vi "Main.vi"(11 "Module Admin":refnum<class "Delacor_lib_QMH_Module Admin.lvclass">) -> ()   [LabVIEW 2022 SP3, in "Server.lvlib"]
doc: "This template is based off of the Queued Message Handler design pattern and the Queued Message Handler project template that ships with LabVIEW.\n\nThe main difference is that the queue is private to this module and communication between modules is performed via Broadcast and Request events.\n\nRequest events are wrapped in public API methods and are handled in the Event Handling Loop (EHL) of this VI. Any module can register for Broadcast events sent by this module. The EHL generates messages based on user interface actions.\n\nThe Message Handling Loop (MHL) processes messages generated by the EHL, or by other messages. The messages are string values, so new messages can be added easily to the Message Cases case structure in the MHL. Each message cluster can also provide an optional value for Message Data, which is a variant that can be converted to whatever message-specific data is required.\n_____\nBased on DQMH Project Template 6.1.0.94."
uses:
  Server.lvlib
  <vilib>/Delacor/Delacor QMH/Libraries/Module Admin_class/Delacor_lib_QMH_Module Admin.lvclass
  Module Data--cluster.ctl
  <vilib>/Delacor/Delacor QMH/Libraries/Message Queue_class/Delacor_lib_QMH_Message Queue.lvclass/Delacor_lib_QMH_Message Queue.ctl
  Stop Argument--cluster.ctl
  <vilib>/Delacor/Delacor QMH/Libraries/Module Admin_class/Delacor_lib_QMH_Module Admin.lvclass/Delacor_lib_QMH_Module Admin.ctl
  <vilib>/Utility/miscctls.llb/LVPointTypeDef.ctl
  <vilib>/Delacor/Delacor QMH/Libraries/Message Queue_class/Delacor_lib_QMH_Enqueue Message (Single).vi
  <vilib>/Delacor/Delacor QMH/Libraries/Module Admin_class/Delacor_lib_QMH_Get External Launch.vi
  <vilib>/Utility/error.llb/Error Cluster From Error Code.vi
  <vilib>/ErrorRing/Error Ring.xnode
  <vilib>/Delacor/Delacor QMH/Libraries/Message Queue_class/Delacor_lib_QMH_Message Queue.lvclass
  User 1/User 1.lvlib
  User 2/User 2.lvlib
panel:
  in  "Launch User 2":bool
  out "error out":errorcluster
  out "Status":string
  in  "Simulate MHL Error":bool
  in  "Simulate EHL Error":bool
  # "Other QMH Modules communicate with this Module via its Public API (wrappers for its Request Events).\n\nThis Module communicates with other Modules via its Broadcast Events.\nAny module that wants to get these messages, just registers for this module's Broadcast events."
  # "This template is for the Delacor Modified Queued Message Handler design pattern.\n\nSee the block diagram for more information on how to use this template."
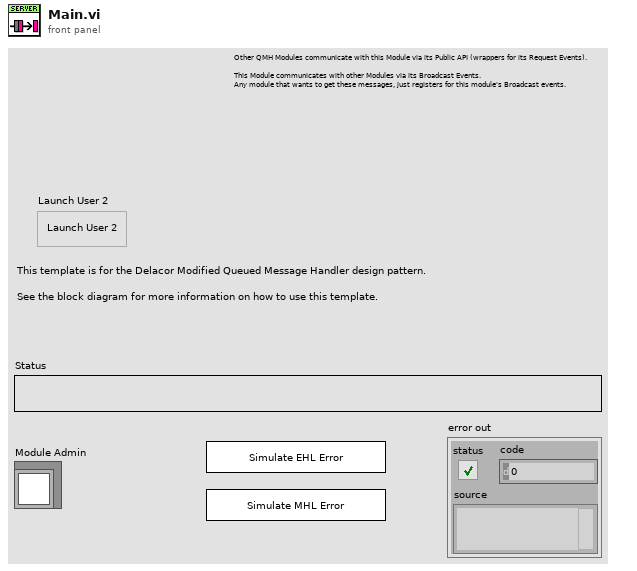
[diagram p1: front panel]
types:
  T1 = typedef "Server.lvlib/Request Events--cluster.ctl" = cluster{"Stop Module":refnum<user-event>, "Show Panel":refnum<user-event>, "Hide Panel":refnum<user-event>, "Get Module Execution Status":refnum<user-event>, "Show Diagram":refnum<user-event>}
  T2 = typedef "User 1.lvlib/Broadcast Events--cluster.ctl" = cluster{"Module Did Init":refnum<user-event>, "Status Updated":refnum<user-event>, "Error Reported":refnum<user-event>, "Module Did Stop":refnum<user-event>, "Update Module Execution Status":refnum<user-event>, "Message was sent":refnum<user-event>}
  T3 = typedef "User 2.lvlib/Broadcast Events--cluster.ctl" = cluster{"Module Did Init":refnum<user-event>, "Status Updated":refnum<user-event>, "Error Reported":refnum<user-event>, "Module Did Stop":refnum<user-event>, "Update Module Execution Status":refnum<user-event>, "Message was sent":refnum<user-event>}
  T4 = typedef "Server.lvlib/Module Data--cluster.ctl" = cluster{"Status":string}
  T5 = enum32{"invalid lock state", "Not Locked", "Locked (No Password)", "Password-protected"}
  T6 = typedef "Server.lvlib/Stop Argument--cluster.ctl" = cluster{"Origin":string, "Exit via Stop Module Req?":bool, "Wait for Module to stop?":bool}
  T7 = typedef "LVPointTypeDef.ctl" = cluster{"Horizontal":i16, "Vertical":i16}
  T8 = enum32{"Invalid", "Standard", "Closed", "Hidden", "Minimized", "Maximized"}
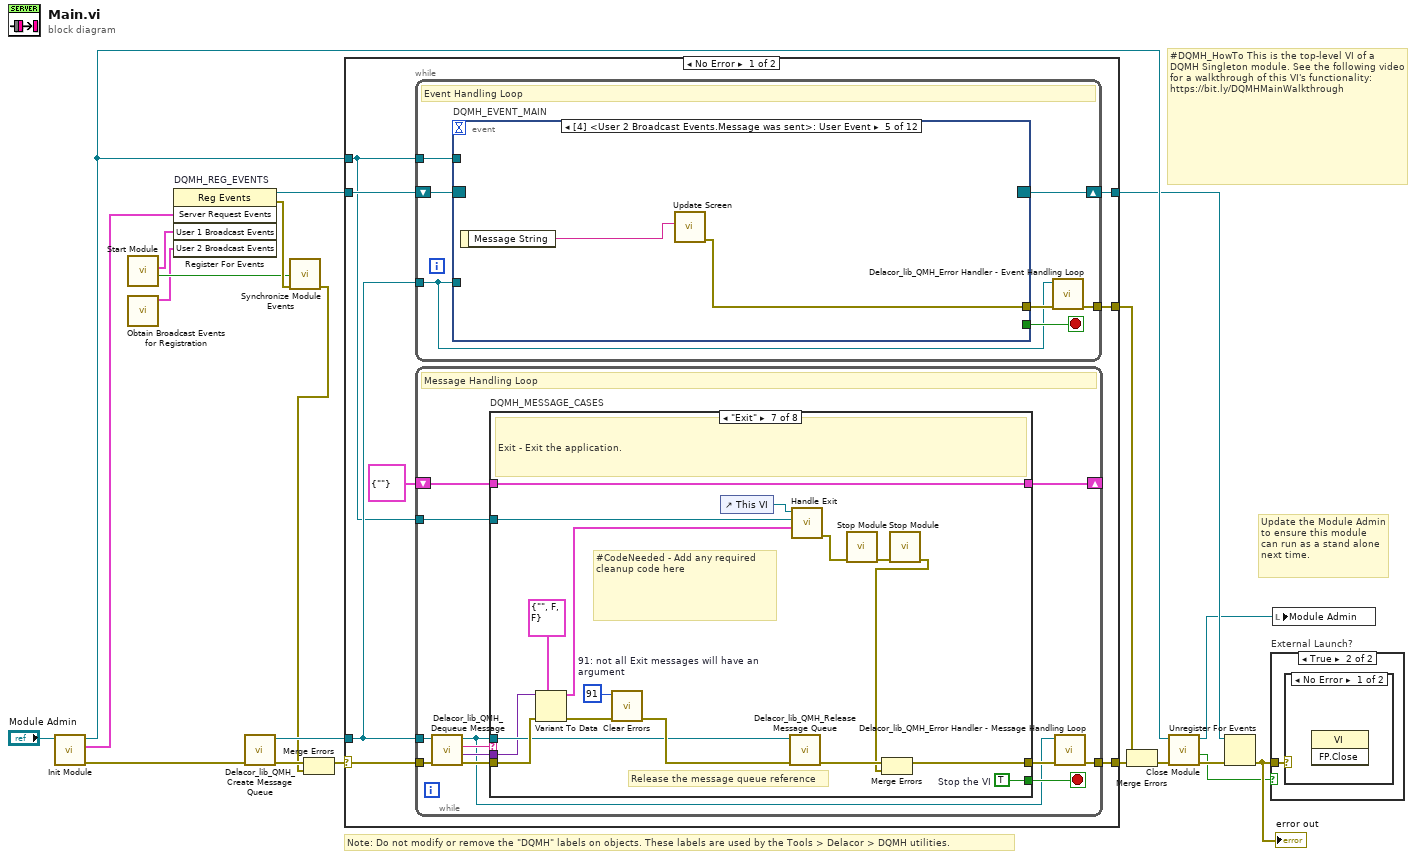
[diagram p0: block diagram]
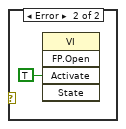
[diagram p3: hidden frame]
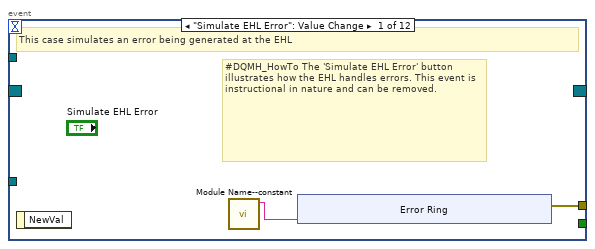
[diagram p4: hidden frame]
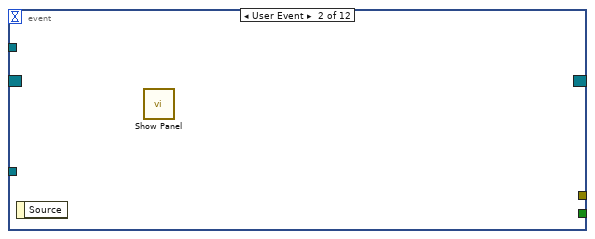
[diagram p5: hidden frame]
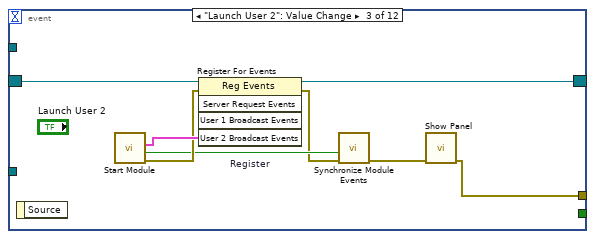
[diagram p6: hidden frame]
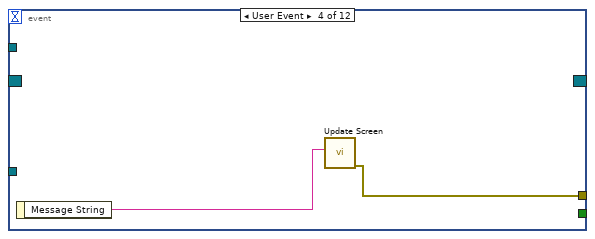
[diagram p7: hidden frame]
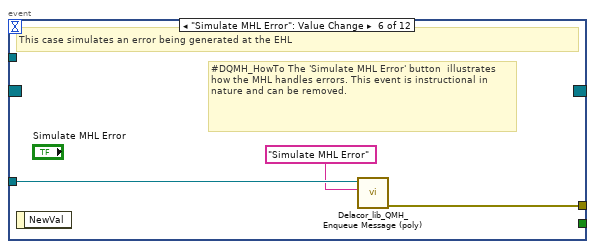
[diagram p8: hidden frame]
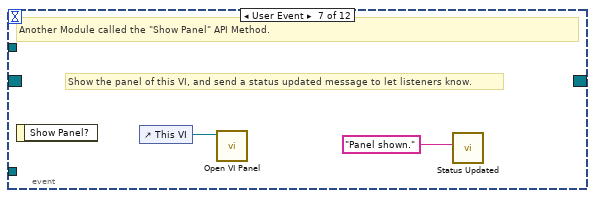
[diagram p9: hidden frame]
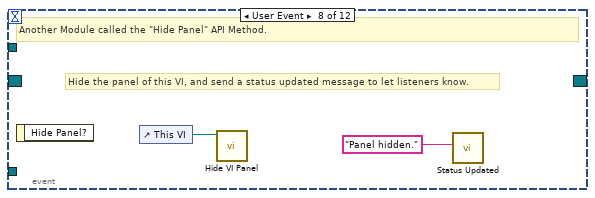
[diagram p10: hidden frame]
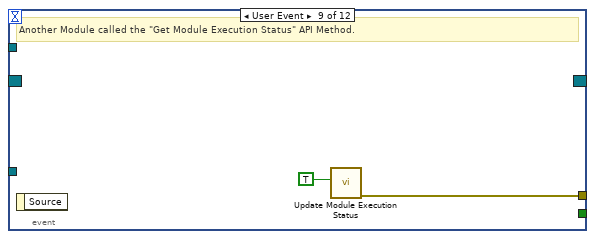
[diagram p11: hidden frame]
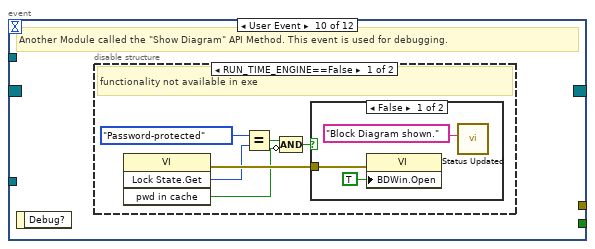
[diagram p12: hidden frame]
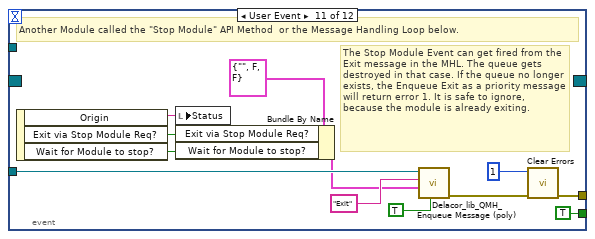
[diagram p15: hidden frame]
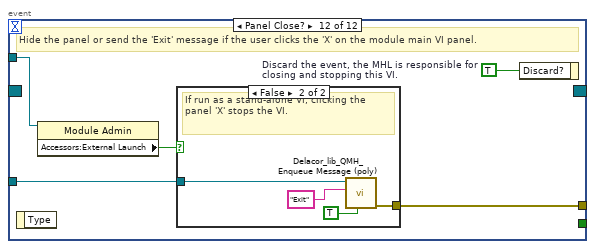
[diagram p16: hidden frame]
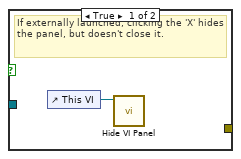
[diagram p17: hidden frame]
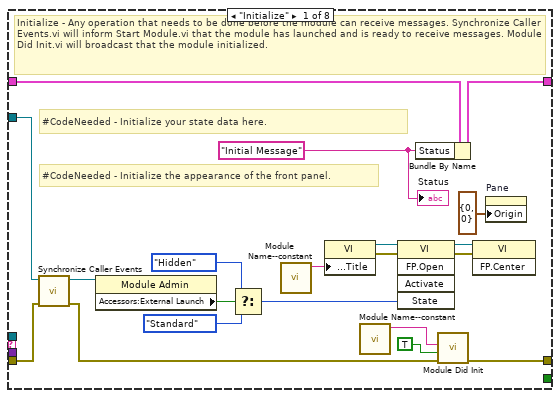
[diagram p18: hidden frame]
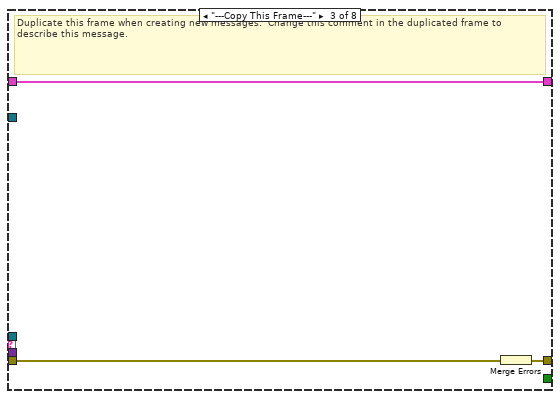
[diagram p20: hidden frame]
diagram:
  # "#DQMH_HowTo This is the top-level VI of a DQMH Singleton module. See the following video for a walkthrough of this VI's functionality: https://bit.ly/DQMHMainWalkthrough"
  # "Note: Do not modify or remove the \"DQMH\" labels on objects. These labels are used by the Tools > Delacor > DQMH utilities."
  # "Update the Module Admin to ensure this module can run as a stand alone next time."
  n1 = call "Init Module.vi"("Singleton Module Admin in"="Module Admin") -> ("error out"=w20:errorcluster, "Server Request Events"=w10:T1, "Singleton Module Admin out"=w13:refnum<class "Delacor_lib_QMH_Module Admin.lvclass">)  [unwired: 8 in]
  n2 = call "Start Module.vi"() -> ("Wait for Event Sync?"=w2:bool, "User 1 Broadcast Events"=w5:T2)  [unwired: 8 in, 2 out]
  n3 = call "Obtain Broadcast Events for Registration.vi"() -> ("User 2 Broadcast Events"=w1:T3)  [unwired: 9 in, 2 out]
  n4 = register-events "DQMH_REG_EVENTS"(w10, w5, w1) -> (reference out=w11:refnum<event-registration>, error out=w4:errorcluster)  [unwired: 2 in]
  n5 = call <vilib>:"Delacor_lib_QMH_Create Message Queue.vi"("error in"=w20) -> ("error out"=w15:errorcluster, "Message Queue"=w9:refnum<class "Delacor_lib_QMH_Message Queue.lvclass">)  [unwired: 9 in]
  n6 = call "Synchronize Module Events.vi"("error in"=w4, "Wait for Event Sync?"=w2) -> ("error out"=w3:errorcluster)  [unwired: 9 in]
  n7 = Merge Errors(w15, w3) -> (w14:errorcluster)
  n8 = case shown="No Error" w14 {
    selector: w14 -> [w27 w198]
    tunnel: [w29 w197] -> w21
    tunnel: [w26 w203] -> w12
    tunnel: w11 -> [w24 w203]
    tunnel: w9 -> [w23 w196]
    tunnel: [w28 _] -> w18
    tunnel: w13 -> [w22 w199]
    frame No Error {
      n9 = while {
        tunnel: w23 -> [w30]
        shift-right: [w33] -> w26
        shift-left: w24 -> [w34]
        tunnel: [w35] -> w28
        tunnel: w22 -> [w31]
        stop <- w32 stop-if-true
        # "Event Handling Loop"
        n10 = event "DQMH_EVENT_MAIN" shown="[4] <User 2 Broadcast Events.Message was sent>: User Event" {
          selector: w34 -> [_ _ w53 _ _ _ _ _ _ _ _ _]
          dyn-events: [_ _ w52 _ _ _ _ _ _ _ _ _] -> w33
          timeout: _ -> [_ _ _ _ _ _ _ _ _ _ _ _]
          tunnel: [_ _ _ _ _ _ _ _ _ _ TRUE ("Discard?") _] -> w32
          tunnel: w30 -> [_ _ _ _ _ w59 _ _ _ _ w83 w90]
          tunnel: [w38 _ w46 w54 w56 w60 _ _ w66 _ w86 w92] -> w36
          tunnel: w31 -> [_ _ _ _ _ _ _ _ _ _ _ w89]
          event "Simulate EHL Error": Value Change {
            # "#DQMH_HowTo The 'Simulate EHL Error' button  illustrates how the EHL handles errors. This event is instructional in nature and can be removed."
            # "This case simulates an error being generated at the EHL"
            n11 = event-data() -> ()  [unwired: 1 in, 1 out]
            n12 = call "Module Name--constant.vi"() -> ("Module Name"=w37:string)  [unwired: 11 in]
            n13 = xnode "Error Ring"("parameter 0"=w37) -> ("error out"=w38:errorcluster)
          }
          event User Event {
            n14 = event-data() -> ()  [unwired: 1 in, 1 out]
            n15 = call "Show Panel.vi"() -> ()  [unwired: 11 in, 1 out]
          }
          event "Launch User 2": Value Change {
            n16 = event-data() -> ()  [unwired: 1 in, 1 out]
            n17 = call "Start Module.vi"() -> ("error out"=w50:errorcluster, "Wait for Event Sync?"=w49:bool, "User 2 Broadcast Events"=w51:T3)  [unwired: 8 in, 1 out]
            n18 = register-events "Register"(reference=w53, error in=w50, w51) -> (reference out=w52:refnum<event-registration>, error out=w48:errorcluster)  [unwired: 2 in]
            n19 = call "Synchronize Module Events.vi"("error in"=w48, "Wait for Event Sync?"=w49) -> ("error out"=w47:errorcluster)  [unwired: 9 in]
            n20 = call "Show Panel.vi"("error in (no error)"=w47) -> ("error out"=w46:errorcluster)  [unwired: 10 in]
          }
          event User Event {
            n21 = event-data() -> ("Message String"=w55:string)  [unwired: 1 in]
            n22 = call "Update Screen.vi"("Message"=w55) -> ("error out"=w54:errorcluster)  [unwired: 10 in]
          }
          event User Event {
            n23 = event-data() -> ("Message String"=w57:string)  [unwired: 1 in]
            n24 = call "Update Screen.vi"("Message"=w57) -> ("error out"=w56:errorcluster)  [unwired: 10 in]
          }
          event "Simulate MHL Error": Value Change {
            # "#DQMH_HowTo The 'Simulate MHL Error' button  illustrates how the MHL handles errors. This event is instructional in nature and can be removed."
            # "This case simulates an error being generated at the EHL"
            n25 = event-data() -> ()  [unwired: 1 in, 1 out]
            n26 = call-poly <vilib>:"Delacor_lib_QMH_Enqueue Message (poly).vi"("Message"="Simulate MHL Error", "Message Queue in"=w59) -> ("error out"=w60:errorcluster)  [unwired: 8 in, 1 out]
          }
          event User Event {
            # "Show the panel of this VI, and send a status updated message to let listeners know."
            # "Another Module called the \"Show Panel\" API Method."
            n27 = event-data() -> ()  [unwired: 1 in, 1 out]
            n28 = control-ref of="This VI"() -> (w62:refnum<vi>)
            n29 = call "Open VI Panel.vi"("VI"=w62) -> ()  [unwired: 10 in, 1 out]
            n30 = call "Status Updated.vi"("Status"="Panel shown." ("format string")) -> ()  [unwired: 10 in, 1 out]
          }
          event User Event {
            # "Hide the panel of this VI, and send a status updated message to let listeners know."
            # "Another Module called the \"Hide Panel\" API Method."
            n31 = event-data() -> ()  [unwired: 1 in, 1 out]
            n32 = control-ref of="This VI"() -> (w64:refnum<vi>)
            n33 = call "Hide VI Panel.vi"("VI"=w64) -> ()  [unwired: 10 in, 1 out]
            n34 = call "Status Updated.vi"("Status"="Panel hidden." ("format string")) -> ()  [unwired: 10 in, 1 out]
          }
          event User Event {
            # "Another Module called the \"Get Module Execution Status\" API Method."
            n35 = event-data() -> ()  [unwired: 1 in, 1 out]
            n36 = call "Update Module Execution Status.vi"("Running?"=TRUE) -> ("error out"=w66:errorcluster)  [unwired: 10 in]
          }
          event User Event {
            # "Another Module called the \"Show Diagram\" API Method. This event is used for debugging."
            n37 = event-data() -> ()  [unwired: 1 in, 1 out]
            n38 = disable-structure shown="RUN_TIME_ENGINE==False" {
              frame condition #0 (active) {
                # "functionality not available in exe"
                n39 = invoke class="VI" method="Lock State.Get"() -> (error out=w72:errorcluster, "Get Lock State"=w71:T5, "pwd in cache"=w68:bool)  [unwired: 4 in, 1 out]
                n40 = Equal?(x=T5."Password-protected", y=w71) -> (x = y?=w69:bool)
                n41 = Compound Arithmetic op=AND(w69, invert w68) -> (w67:bool)
                n42 = case shown="False" w67 {
                  tunnel: w72 -> [w75 _]
                  frame False {
                    n43 = property class="VI"(error in=w75, "BDWin.Open"=TRUE ("Block Diagram Window:Open")) -> ()  [unwired: 1 in, 2 out]
                    n44 = call "Status Updated.vi"("Status"="Block Diagram shown." ("format string")) -> ()  [unwired: 10 in, 1 out]
                  }
                  frame True {
                    # "Password-protected VI, and the password is not in the cache. Do not show the diagram."
                  }
                }
              }
              frame condition #1 {
              }
            }
          }
          event User Event {
            # "The Stop Module Event can get fired from the Exit message in the MHL. The queue gets destroyed in that case. If the queue no longer exists, the Enqueue Exit as a priority message will return error 1. It is safe to ignore, because the module is already exiting."
            # "Another Module called the \"Stop Module\" API Method  or the Message Handling Loop below."
            n45 = event-data() -> ("Origin"=w82:string, "Exit via Stop Module Req?"=w78:bool, "Wait for Module to stop?"=w77:bool)  [unwired: 1 in]
            n46 = local write "Status"(w82) -> ()
            n47 = Bundle By Name(cluster=T6 {"Origin"="", "Exit via Stop Module Req?"=FALSE, "Wait for Module to stop?"=FALSE} ("Stop Argument"), "Exit via Stop Module Req?"=w78, "Wait for Module to stop?"=w77) -> (w76:T6)
            n48 = call-poly <vilib>:"Delacor_lib_QMH_Enqueue Message (poly).vi"("Priority Message? (F)"=TRUE, "Message Data"=w76, "Message"="Exit", "Message Queue in"=w83) -> ("error out"=w87:errorcluster)  [unwired: 6 in, 1 out]
            n49 = call <vilib>:"Clear Errors.vi"("error in (no error)"=w87, "specific error code to clear (0: all)"=1) -> ("error out"=w86:errorcluster)  [unwired: 4 in, 1 out]
          }
          event Panel Close? {
            w91 = TRUE  # Discard the event, the MHL is responsible for closing and stopping this VI.
            # "Hide the panel or send the 'Exit' message if the user clicks the 'X' on the module main VI panel."
            n50 = event-data() -> ()  [unwired: 1 in, 1 out]
            n51 = property class="Module Admin"(reference=w89) -> ("Accessors:External Launch"=w88:bool)  [unwired: 1 in, 2 out]
            n52 = case shown="False" w88 {
              tunnel: w90 -> [_ w96]
              tunnel: [_ w97] -> w92
              frame True {
                # "If externally launched, clicking the 'X' hides the panel, but doesn't close it."
                n53 = control-ref of="This VI"() -> (w93:refnum<vi>)
                n54 = call "Hide VI Panel.vi"("VI"=w93) -> ()  [unwired: 10 in, 1 out]
              }
              frame False {
                # "If run as a stand-alone VI, clicking the panel 'X' stops the VI."
                n55 = call-poly <vilib>:"Delacor_lib_QMH_Enqueue Message (poly).vi"("Priority Message? (F)"=TRUE, "Message"="Exit", "Message Queue in"=w96) -> ("error out"=w97:errorcluster)  [unwired: 7 in, 1 out]
              }
            }
            n56 = event-data("Discard?"=w91) -> ()  [unwired: 1 in, 1 out]
          }
        }
        n57 = call-dynamic "Delacor_lib_QMH_Error Handler - Event Handling Loop.vi"("error in"=w36, "Message Queue in"=w30) -> ("dup error in"=w35:errorcluster)  [unwired: 8 in, 1 out]
      }
      n58 = while {
        tunnel: w23 -> [w100]
        shift-right: [w104] -> _
        shift-left: T4 {"Status"=""} ("Data Cluster") -> [w105]
        tunnel: w27 -> [w108]
        tunnel: [w106] -> w29
        tunnel: w22 -> [w98]
        stop <- w103 stop-if-true
        # "Message Handling Loop"
        n59 = call-dynamic "Delacor_lib_QMH_Dequeue Message.vi"("error in"=w108, "Message Queue in"=w100) -> ("error out"=w107:errorcluster, "Message Data"=w101:variant, "Message"=w102:string, "Message Queue out"=w99:refnum<class "Delacor_lib_QMH_Message Queue.lvclass">)  [unwired: 6 in]
        n60 = case "DQMH_MESSAGE_CASES" shown="\"Exit\"" w102 {
          selector: w102 -> [_ _ _ _ _ _ _ w183]
          tunnel: w99 -> [_ _ _ _ _ w151 w176 _]
          tunnel: w107 -> [w127 w131 w134 w136 w141 w158 w181 w185]
          tunnel: [w125 w131 w133 w136 w140 w154 w178 w186] -> w109
          tunnel: w105 -> [w116 w130 w132 w135 w138 w153 w175 w184]
          tunnel: [w115 w130 w132 w135 w138 w153 w175 w184] -> w104
          tunnel: [_ _ _ _ _ _ w174 _] -> w103
          tunnel: w101 -> [_ _ _ _ _ w152 w173 _]
          tunnel: w98 -> [w117 _ _ _ _ w150 w168 _]
          frame "Initialize" {
            w111 = "Initial Message" ("Initial Message")
            # "#CodeNeeded - Initialize the appearance of the front panel."
            # "#CodeNeeded - Initialize your state data here."
            # "Initialize - Any operation that needs to be done before the module can receive messages. Synchronize Caller Events.vi will inform Start Module.vi that the module has launched and is ready to receive messages. Module Did Init.vi will broadcast that the module initialized."
            n61 = call "Synchronize Caller Events.vi"("error in (no error)"=w127, "Singleton Module Admin in"=w117) -> ("error out"=w126:errorcluster, "Singleton Module Admin out"=w112:refnum<class "Delacor_lib_QMH_Module Admin.lvclass">)  [unwired: 8 in]
            n62 = property class="Module Admin"(reference=w112) -> ("Accessors:External Launch"=w121:bool)  [unwired: 1 in, 2 out]
            n63 = Select(t=T8."Hidden" ("State"), s=w121, f=T8."Standard" ("State")) -> (s? t:f=w118:T8)
            n64 = call "Module Name--constant.vi"() -> ("Module Name"=w124:string)  [unwired: 11 in]
            n65 = property class="VI"("Front Panel.Title"=w124) -> (reference out=w123:refnum<vi>, error out=w129:errorcluster)  [unwired: 2 in]
            n66 = call "Module Name--constant.vi"() -> ("Module Name"=w113:string)  [unwired: 11 in]
            n67 = invoke class="VI" method="FP.Open"(reference=w123, error in=w129, "State"=w118) -> (reference out=w122:refnum<vi>, error out=w128:errorcluster)  [unwired: 2 in, 3 out]
            n68 = Bundle By Name(cluster=w116, "Status"=w111) -> (w115:T4)
            n69 = call "Module Did Init.vi"("error in (no error)"=w126, "Initialized?"=TRUE, "Origin"=w113) -> ("error out"=w125:errorcluster)  [unwired: 8 in]
            n70 = invoke class="VI" method="FP.Center"(reference=w122, error in=w128) -> ()  [unwired: 1 in, 3 out]
            n71 = property on="Pane" class="Pane"("Origin"=T7 {"Horizontal"=0, "Vertical"=0}) -> ()  [unwired: 2 in, 2 out]
            "Status" <- w111
          }
          frame "---Module Specific---" {
            # "Separator -- The following cases handle messages specific to this Module."
          }
          frame "---Copy This Frame---" {
            # "Duplicate this frame when creating new messages.  Change this comment in the duplicated frame to describe this message."
            n72 = Merge Errors(w134) -> (w133:errorcluster)
          }
          frame "---Exit and Error Handling---" {
            # "Separator - The following cases handle errors and exit messages."
          }
          frame "Simulate MHL Error" {
            # "#DQMH_HowTo The 'Simulate MHL Error' button  illustrates how the MHL handles errors. This event is instructional in nature and can be removed."
            # "Simulate an error occurring at the MHL"
            n73 = call "Module Name--constant.vi"() -> ("Module Name"=w137:string)  [unwired: 11 in]
            n74 = xnode "Error Ring"("parameter 0"=w137) -> ("error out"=w139:errorcluster)
            n75 = Merge Errors(w141, w139) -> (w140:errorcluster)
          }
          frame "Error" {
            # "#CodeRecommended - If you ever change the name of this \"Error\" message, you'll need to update the name in the Check Loop Error.vi as well."
            # "#CodeRecommended - If the module is running in standalone mode (External Launch = FALSE), this code will pop up an error dialog and call the 'Exit' message if an error occurs. Add more fine-grained error handling here."
            # "Error - Check the error message data and respond accordingly. This message is sent by the \"Error Handler\" VIs at the end of each loop in this application."
            n76 = property class="Module Admin"(reference=w150) -> ("Accessors:External Launch"=w149:bool)  [unwired: 1 in, 2 out]
            n77 = Variant To Data(error in=w158, type=errorcluster {"status"=FALSE, "code"=0, "source"=""} ("error constant"), Variant=w152) -> (data=w159:errorcluster, error out=w156:errorcluster)
            n78 = call "Error Reported.vi"("Error"=w159) -> ()  [unwired: 10 in, 1 out]
            n79 = case shown="False" w149 {
              tunnel: [w164 _] -> w155
              tunnel: w151 -> [w162 _]
              tunnel: w159 -> [w163 _]
              frame False {
                # "If the module is running standalone, then pop up an error dialog and call the \"Exit\" message."
                n80 = call <vilib>:"Simple Error Handler.vi"("error in (no error)"=w163) -> ()  [unwired: 4 in, 5 out]
                n81 = call-poly <vilib>:"Delacor_lib_QMH_Enqueue Message (poly).vi"("Priority Message? (F)"=TRUE, "Message"="Exit", "Message Queue in"=w162) -> ("error out"=w164:errorcluster)  [unwired: 7 in, 1 out]
              }
              frame True {
                # "If the module was launched externally, calling the Error Reported broadcast VI is the only action performed by the \"Error\" message. The module's caller can then process the error appropriately."
              }
            }
            n82 = Merge Errors(w156, w155) -> (w154:errorcluster)
            n83 = local write "error out"(w154) -> ()
          }
          frame "Exit" {
            w172 = 91  # 91: not all Exit messages will have an argument
            w174 = TRUE  # Stop the VI
            # "Release the message queue reference"
            # "#CodeNeeded - Add any required cleanup code here"
            # "Exit - Exit the application."
            n84 = Variant To Data(error in=w181, type=T6 {"Origin"="", "Exit via Stop Module Req?"=FALSE, "Wait for Module to stop?"=FALSE} ("Stop Argument"), Variant=w173) -> (data=w170:T6, error out=w177:errorcluster)
            n85 = call <vilib>:"Clear Errors.vi"("error in (no error)"=w177, "specific error code to clear (0: all)"=w172) -> ("error out"=w180:errorcluster)  [unwired: 4 in, 1 out]
            n86 = control-ref of="This VI"() -> (w169:refnum<vi>)
            n87 = call-dynamic "Delacor_lib_QMH_Release Message Queue.vi"("error in"=w180, "Message Queue"=w176) -> ("error out"=w179:errorcluster)  [unwired: 9 in]
            n88 = call "Handle Exit.vi"("Stop Argument"=w170, "Admin in"=w168, "VI reference"=w169) -> ("error out"=w167:errorcluster)  [unwired: 7 in, 1 out]
            n89 = call "Stop Module.vi"("error in"=w167) -> ("error out"=w166:errorcluster)  [unwired: 10 in]
            n90 = call "Stop Module.vi"("error in"=w166) -> ("error out"=w165:errorcluster)  [unwired: 10 in]
            n91 = Merge Errors(w179, w165) -> (w178:errorcluster)
          }
          frame Default {
            # "'Default' case only runs if there is a message that isn't defined in any of the other cases.  Output a programming error."
            n92 = call "Module Name--constant.vi"() -> ("Module Name"=w182:string)  [unwired: 11 in]
            n93 = xnode "Error Ring"("parameter 0"=w183, "parameter 1"=w182) -> ("error out"=w187:errorcluster)
            n94 = Merge Errors(w185, w187) -> (w186:errorcluster)
          }
        }
        n95 = call-dynamic "Delacor_lib_QMH_Error Handler - Message Handling Loop.vi"("error in"=w109, "Message Queue in"=w99) -> ("dup error in"=w106:errorcluster)  [unwired: 8 in, 1 out]
      }
    }
    frame Error {
      # "Synchronize Caller Events.vi will inform Start Module.vi that the module has launched and will let the code calling Start Module.vi register for broadcasts and would permit the caller receive the broadcast that an error occurred at launch time."
      n96 = call-dynamic "Delacor_lib_QMH_Release Message Queue.vi"("error in"=w198, "Message Queue"=w196) -> ("error out"=w197:errorcluster)  [unwired: 9 in]
      n97 = call "Synchronize Caller Events.vi"("Singleton Module Admin in"=w199) -> ("error out"=w204:errorcluster)  [unwired: 9 in, 1 out]
      n98 = call "Module Name--constant.vi"() -> ("Module Name"=w202:string)  [unwired: 11 in]
      n99 = Format Into String(format string="An error occurred during initialization. %s is no longer running.", w202) -> (resulting string=w200:string)  [unwired: 2 in, 1 out]
      n100 = Merge Errors(w197, w204) -> (w205:errorcluster)
      n101 = call "Error Reported.vi"("Additional Information"=w200, "Error"=w205) -> ()  [unwired: 9 in, 1 out]
    }
  }
  n102 = Merge Errors(w18, w21) -> (w17:errorcluster)
  n103 = call "Close Module.vi"("error in (no error)"=w17, "Module Admin in"=w13) -> ("error out"=w19:errorcluster, "External Launch"=w6:bool, "Module Admin out"=w7:refnum<class "Delacor_lib_QMH_Module Admin.lvclass">)  [unwired: 7 in]
  n104 = Unregister For Events(event registration refnum=w12, error in=w19) -> (error out=w16:errorcluster)
  "error out" <- w16
  n105 = case "External Launch?" shown="True" w6 {
    tunnel: w16 -> [_ w206]
    frame False {
    }
    frame True {
      n106 = case shown="No Error" w206 {
        frame No Error {
          n107 = invoke class="VI" method="FP.Close"() -> ()  [unwired: 3 in, 3 out]
        }
        frame Error {
          n108 = invoke class="VI" method="FP.Open"("Activate"=TRUE ("Activate?")) -> ()  [unwired: 4 in, 5 out]
        }
      }
    }
  }
  n109 = local write "Module Admin"(w7) -> ()
